vi "IPI_CalNewXY.vi"(6 "Y in":dbl[](array[numeric]) caption="Y输出", 7 "X in":dbl[](array[numeric]) caption="X输出", 8 "Hel":dbl=-4.6 format="%#_13g", 9 "Ver":dbl=4.0 format="%#_13g", 10 "theta":dbl=-0.02 format="%#_13g", 11 "Step1 XY Pos":string[][](array[string])) -> (0 "添加的数组":string[][](array[string]), 2 "NEW Y":dbl[](array[numeric]), 3 "New X":dbl[](array[numeric]))   [LabVIEW 2015]
uses:
  <vilib>/Analysis/coordinate.llb/2D Cartesian Coordinate Rotation (Array).vi
  <vilib>/Analysis/NI_AALPro.lvlib
panel:
  out "Y Out":dbl[](array[numeric]) caption="Y输出"
  out "X Out":dbl[](array[numeric]) caption="X输出"
  out "x*y":dbl
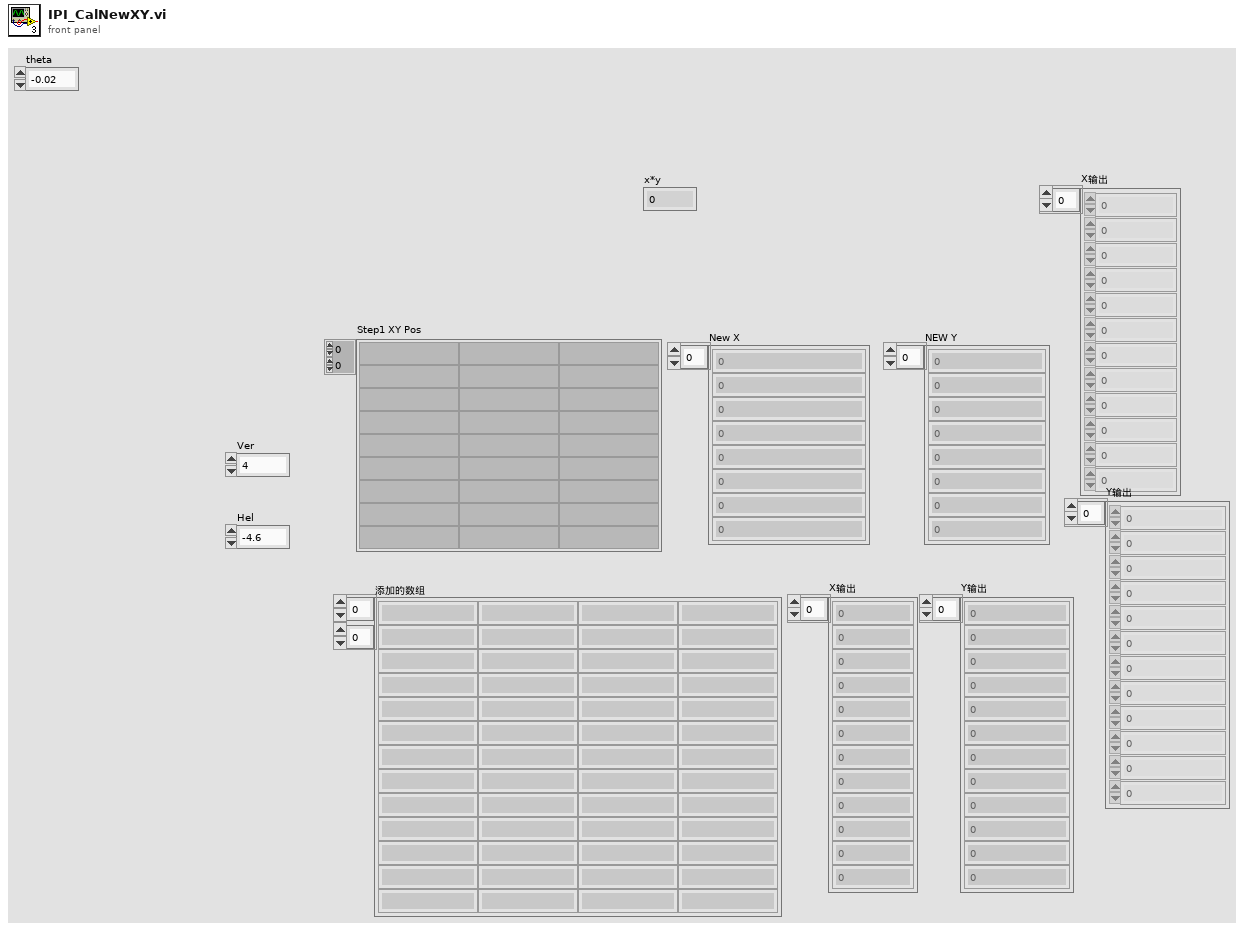
[diagram p1: front panel]
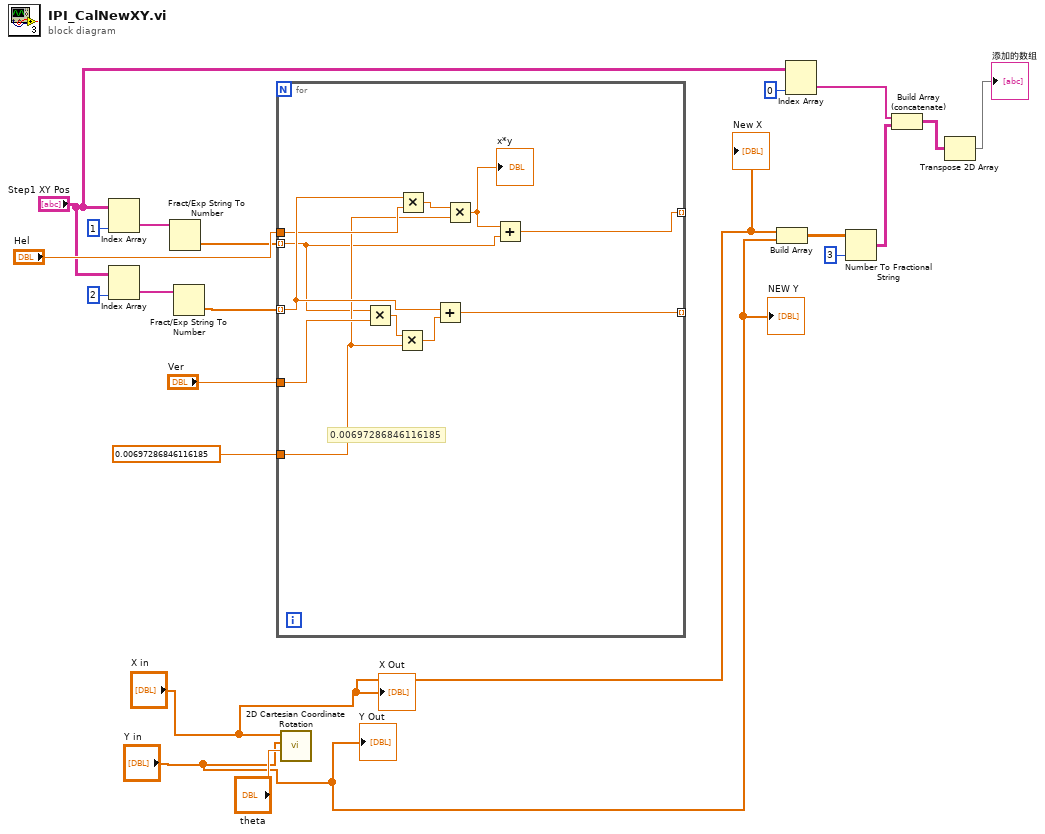
[diagram p0: block diagram]
diagram:
  n1 = Index Array(array="Step1 XY Pos", index (col)=1 ("禁用的索引 (列)")) -> (element=w18:string[])  [unwired: 1 in]
  n2 = Index Array(array="Step1 XY Pos", index (col)=2 ("禁用的索引 (列)")) -> (element=w17:string[])  [unwired: 1 in]
  n3 = Fract/Exp String To Number(string=w18) -> (number=w3:dbl[])  [unwired: 3 in, 1 out]
  n4 = Fract/Exp String To Number(string=w17) -> (number=w5:dbl[])  [unwired: 3 in, 1 out]
  n5 = for {
    tunnel: w3 -> [w22] mode=indexing
    tunnel: w5 -> [w27] mode=indexing
    tunnel: "Ver" -> [w31]
    tunnel: 0.00697286846116185 ("y") -> [w24]
    tunnel: [w28] -> _ mode=indexing
    tunnel: "Hel" -> [w26]
    tunnel: [w21] -> _ mode=indexing
    # "0.00697286846116185"
    n6 = Multiply(x=w22, y=w31) -> (x*y=w30:dbl)
    n7 = Multiply(x=w30, y=w24) -> (x*y=w29:dbl)
    n8 = Multiply(x=w27, y=w26) -> (x*y=w25:dbl)
    n9 = Add(x=w27, y=w29) -> (x+y=w28:dbl)
    n10 = Multiply(x=w25, y=w24) -> (x*y=w23:dbl)
    "x*y" <- w23
    n11 = Add(x=w23, y=w22) -> (x+y=w21:dbl)
  }
  n12 = call-poly <vilib>:"2D Cartesian Coordinate Rotation.vi"("theta"="theta", "Y"="Y in", "X"="X in") -> ()  [unwired: 6 in, 3 out]
  n13 = Build Array("X in", "Y in") -> (w11:dbl[][])
  n14 = Index Array(array="Step1 XY Pos", index (col)=0 ("禁用的索引 (列)")) -> (element=w9:string[])  [unwired: 1 in]
  n15 = Number To Fractional String(number=w11, precision (6)=i16 3 ("精度(6)")) -> (F-format string=w8:string[][])  [unwired: 2 in]
  n16 = Build Array (concatenate)(w9, w8) -> (w7:string[][])
  n17 = Transpose 2D Array(2D array=w7) -> (transposed array=→"添加的数组":string[][])
  "New X" <- "X in"
  "NEW Y" <- "Y in"
  "X Out" <- "X in"
  "Y Out" <- "Y in"
